vi "isEmpty.vi"(8 "error in (no error)":errorcluster, 11 "xwpfParagraph in":refnum<class "xwpfParagraph.lvclass">) -> (0 "error out":errorcluster, 2 "IsEmpty":bool, 3 "xwpfParagraph out":refnum<class "xwpfParagraph.lvclass">)   [LabVIEW 2017, in "Word_Specific.lvlib" / "xwpfParagraph.lvclass"]
uses:
  xwpfParagraph.lvclass
  xwpfParagraph.lvclass/xwpfParagraph.ctl
  C:/Users/Neo/Desktop/Dev_Tools_BR/LabVIEW_NPOI/src/lib/NPOI 2.1.1/NPOI.OOXML.dll
  lib/NPOI 2.1.1/NPOI.OOXML.dll
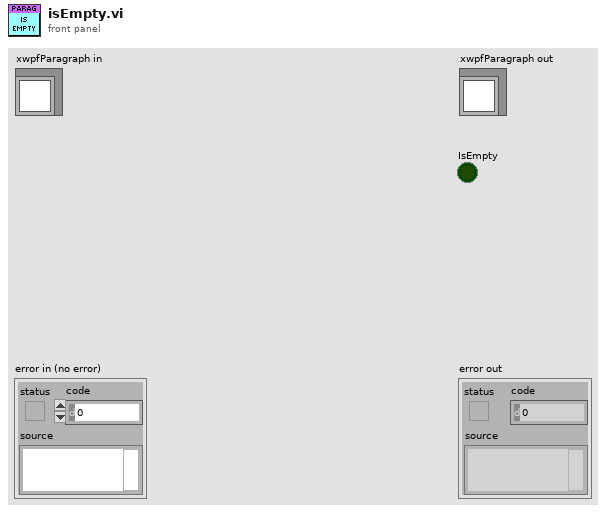
[diagram p1: front panel]
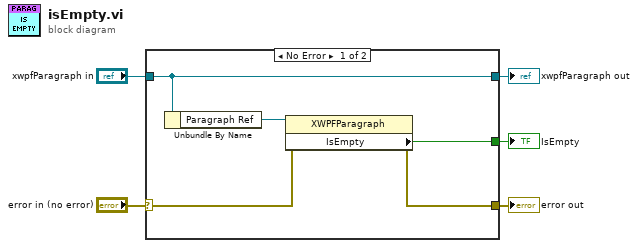
[diagram p0: block diagram]
diagram:
  n1 = case shown="No Error" "error in (no error)" {
    selector: "error in (no error)" -> [w7 w12]
    tunnel: [w6 w12] -> w2
    tunnel: [w10 w11] -> w4
    tunnel: "xwpfParagraph in" -> [w10 w11]
    tunnel: [w9 _] -> w1
    frame No Error {
      n2 = Unbundle By Name(w10) -> ("Paragraph Ref"=w8:refnum<k24>)
      n3 = property class="XWPFParagraph"(reference=w8, error in=w7) -> (error out=w6:errorcluster, "IsEmpty"=w9:bool)  [unwired: 1 out]
    }
    frame Error {
    }
  }
  "error out" <- w2
  "xwpfParagraph out" <- w4
  "IsEmpty" <- w1
